vi "CRYWrap Phase180.vi"(11 "Phase In":dbl[](array[numeric])) -> (3 "Phase Out":dbl[](array[numeric]))   [LabVIEW 2013]
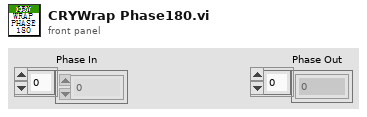
[diagram p1: front panel]
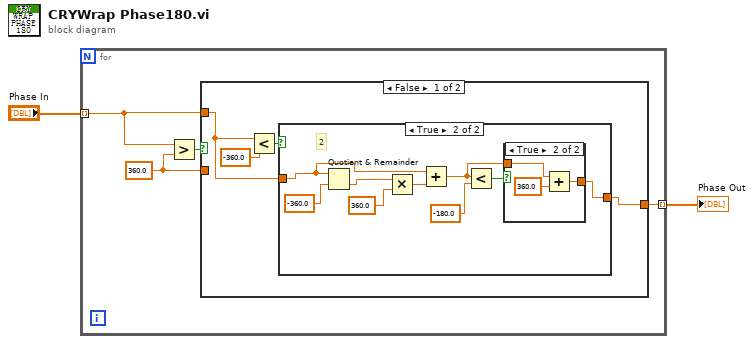
[diagram p0: block diagram]
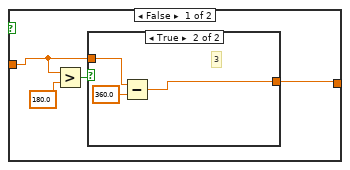
[diagram p2: hidden frame]
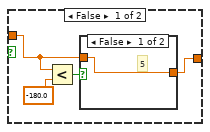
[diagram p3: hidden frame]
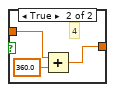
[diagram p4: hidden frame]
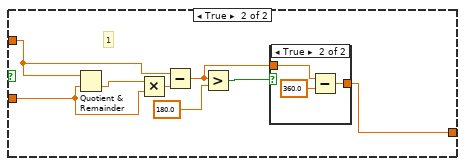
[diagram p6: hidden frame]
diagram:
  n1 = for {
    tunnel: "Phase In" -> [w4] mode=indexing
    tunnel: [w3] -> w1 mode=indexing
    w5 = 360.0 ("y")
    n2 = Greater?(x=w4, y=w5) -> (0:w6:bool)
    n3 = case shown="False" w6 {
      tunnel: w4 -> [w8 w44]
      tunnel: w5 -> [_ w46]
      tunnel: [w7 w40] -> w3
      frame False {
        n4 = Less?(x=w8, y=-360.0) -> (x < y?=w10:bool)
        n5 = case shown="True" w10 {
          tunnel: w8 -> [w12 w33]
          tunnel: [w11 w29] -> w7
          frame False {
            n6 = Greater?(x=w12, y=180.0) -> (0:w13:bool)
            n7 = case shown="True" w13 {
              tunnel: w12 -> [w16 w25]
              tunnel: [w15 w23] -> w11
              frame False {
                n8 = Less?(x=w16, y=-180.0) -> (x < y?=w17:bool)
                n9 = case shown="False" w17 {
                  tunnel: w16 -> [w19 w22]
                  tunnel: [w19 w20] -> w15
                  frame False {
                    # "5"
                  }
                  frame True {
                    # "4"
                    n10 = Add(x=w22, y=360.0) -> (x+y=w20:dbl)
                  }
                }
              }
              frame True {
                # "3"
                n11 = Subtract(x=w25, y=360.0) -> (x-y=w23:dbl)
              }
            }
          }
          frame True {
            # "2"
            n12 = Quotient & Remainder(x=w33, y=-360.0) -> (floor(x/y)=w28:dbl)  [unwired: 1 out]
            n13 = Multiply(x=w28, y=360.0) -> (x*y=w34:dbl)
            n14 = Add(x=w33, y=w34) -> (x+y=w30:dbl)
            n15 = Less?(x=w30, y=-180.0) -> (x < y?=w31:bool)
            n16 = case shown="True" w31 {
              tunnel: w30 -> [w35 w38]
              tunnel: [w35 w36] -> w29
              frame False {
              }
              frame True {
                n17 = Add(x=w38, y=360.0) -> (x+y=w36:dbl)
              }
            }
          }
        }
      }
      frame True {
        # "1"
        n18 = Quotient & Remainder(x=w44, y=w46) -> (floor(x/y)=w39:dbl)  [unwired: 1 out]
        n19 = Multiply(x=w39, y=w46) -> (x*y=w45:dbl)
        n20 = Subtract(x=w44, y=w45) -> (x-y=w41:dbl)
        n21 = Greater?(x=w41, y=180.0) -> (0:w42:bool)
        n22 = case shown="True" w42 {
          tunnel: w41 -> [w47 w50]
          tunnel: [w47 w48] -> w40
          frame False {
          }
          frame True {
            n23 = Subtract(x=w50, y=360.0) -> (x-y=w48:dbl)
          }
        }
      }
    }
  }
  "Phase Out" <- w1
